vi "例5-6.vi"() -> ()   [LabVIEW 2019]
uses:
  <vilib>/DAQmx/read.llb/DAQmx Read (Digital 1D Bool NChan 1Samp 1Line).vi
  <vilib>/DAQmx/create/channels.llb/DAQmx Create Channel (DI-Digital Input).vi
  <vilib>/DAQmx/miscellaneous.llb/DAQmx Fill In Error Info.vi
panel:
  out "I/O线状态":bool[](array[boolean])
  in  "I/O线":tag[](array[tag])
  in  "停止":bool
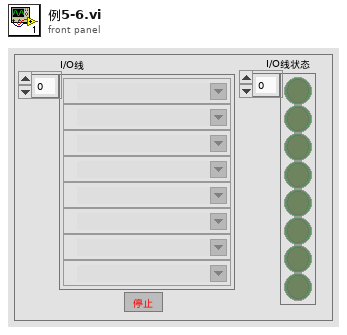
[diagram p1: front panel]
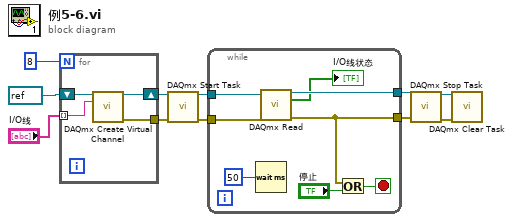
[diagram p0: block diagram]
diagram:
  n1 = for {
    N: 8 -> [_]
    shift-right: [w14] -> w9
    shift-left: refnum<k21> refnum ("task in") -> [w15]
    tunnel: [w13] -> w7
    tunnel: "I/O线" -> [w12] mode=indexing
    n2 = call-poly <vilib>:"DAQmx Create Virtual Channel.vi"("task in"=w15, "lines"=w12) -> ("task out"=w14:refnum<k21>, "error out"=w13:errorcluster)  [unwired: 12 in]
  }
  n3 = call <vilib>:"DAQmx Start Task.vi"("task/channels in"=w9, "error in"=w7) -> ("task out"=w8:refnum<k21>, "error out"=w6:errorcluster)  [unwired: 12 in]
  n4 = while {
    tunnel: w8 -> [w23]
    tunnel: w6 -> [w22]
    tunnel: [w20] -> w3
    tunnel: [w19] -> w2
    stop <- w17 stop-if-true
    n5 = Wait (ms)(milliseconds to wait=50) -> ()  [unwired: 1 out]
    n6 = call-poly <vilib>:"DAQmx Read.vi"("task/channels in"=w23, "error in"=w22) -> ("task out"=w20:refnum<k21>, "data"=→"I/O线状态":bool[], "error out"=w19:errorcluster)  [unwired: 11 in]
    n7 = Or(x=w19, y="停止") -> (x .or. y?=w17:bool)
  }
  n8 = call <vilib>:"DAQmx Stop Task.vi"("task/channels in"=w3, "error in"=w2) -> ("task out"=w5:refnum<k21>, "error out"=w4:errorcluster)  [unwired: 12 in]
  n9 = call <vilib>:"DAQmx Clear Task.vi"("task in"=w5, "error in"=w4) -> ()  [unwired: 13 in, 1 out]
